vi "Enable Signal Display.vi"(8 "error in (no error)":errorcluster, 9 "Enable Signal Display (T: Enable)":bool=TRUE, 10 "Signal Name (0: Channel 1)":i32(ring) items=["Channel 1"=0, "Channel 2"=1, "Channel 3"=2, "Channel 4"=3, "Function"=4, "Serial Bus 1"=7, "Serial Bus 2"=8, "Digital Bus Low"=9, "Digital Bus High"=10, "Digital Bus 1"=11, "Digital Bus 2"=12, "D0"=13, "D1"=14, "D2"=15, "D3"=16, "D4"=17, "D5"=18, "D6"=19, "D7"=20, "D8"=21, "D9"=22, "D10"=23, "D11"=24, "D12"=25, "D13"=26, "D14"=27, "D15"=28, "External"=29, "Function 1"=32, "Function 2"=33, "Function 3"=34, "Function 4"=35, "Math 1"=36, "Math 2"=37, "Math 3"=38, "Math 4"=39, "Math"=40, "FFT"=41, "Analog Bus"=42], 11 "VISA resource name":refnum<visa-resource-name>) -> (0 "error out":errorcluster, 3 "VISA resource name out":refnum<visa-resource-name>)   [LabVIEW 2016, in "Agilent 2000 3000 X-Series.lvlib"]
doc: "Configures the front panel display of signal."
uses:
  Agilent 2000 3000 X-Series.lvlib
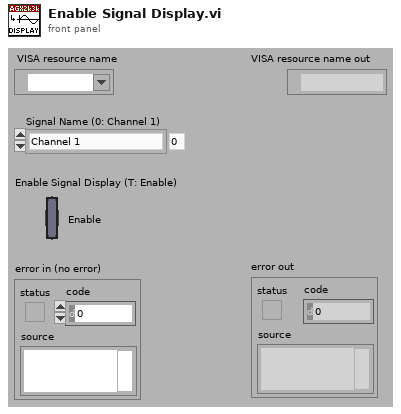
[diagram p1: front panel]
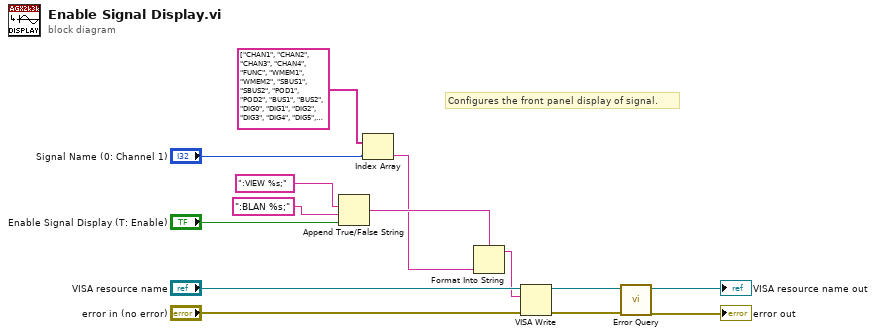
[diagram p0: block diagram]
diagram:
  # "Configures the front panel display of signal."
  n1 = Append True/False String(1:"Enable Signal Display (T: Enable)", 2:":BLAN %s;", 3:":VIEW %s;") -> (0:w5:string)  [unwired: 1 out]
  n2 = Index Array(array=string[] ["CHAN1", "CHAN2", "CHAN3", "CHAN4", "FUNC", "WMEM1", "WMEM2", "SBUS1", "SBUS2", "POD1", "POD2", "BUS1", "BUS2", "DIG0", "DIG1", "DIG2", "DIG3", "DIG4", "DIG5", "DIG6", "DIG7", "DIG8", "DIG9", "DIG10", "DIG11", "DIG12", "DIG13", "DIG14", "DIG15", "EXT", "LINE", "WGEN", "FUNC1", "FUNC2", "FUNC3", "FUNC4", "MATH1", "MATH2", "MATH3", "MATH4", "MATH", "FFT", "ABUS"], index="Signal Name (0: Channel 1)") -> (element=w2:string)
  n3 = Format Into String(format string=w5, w2) -> (resulting string=w4:string)  [unwired: 2 in, 1 out]
  n4 = VISA Write(VISA resource name="VISA resource name", write buffer=w4, error in (no error)="error in (no error)") -> (VISA resource name out=w12:refnum<visa-resource-name>, error out=w11:errorcluster)  [unwired: 1 out]
  n5 = call "Error Query.vi"("error in (no error)"=w11, "VISA resource name"=w12) -> ("error out"=→"error out":errorcluster, "VISA resource name out"=→"VISA resource name out":refnum<visa-resource-name>)  [unwired: 8 out]
